vi "PathPlanner_IdealStartingState_Equals.vi"(9 "Other IdealStartingState":T1={"VelocityMPS"=0.0, "Rotation"={"VALUE"=0.0, "COS"=1.0, "SIN"=0.0}, "NotNull"=FALSE} {"Rotation"."SIN" format="%13.4f"; "Rotation"."COS" format="%13.4f"; "Rotation"."VALUE" format="%13.4f"}, 11 "IdealStartingState":T1={"VelocityMPS"=0.0, "Rotation"={"VALUE"=0.0, "COS"=1.0, "SIN"=0.0}, "NotNull"=FALSE} {"Rotation"."SIN" format="%13.4f"; "Rotation"."COS" format="%13.4f"; "Rotation"."VALUE" format="%13.4f"}) -> (3 "Equal":bool)   [LabVIEW 2019, in "PathPlanner24.lvlib"]
doc: "Determines if two Ideal Starting State definitions are equal\n\nInputs:\n -- IdealStartingState - cluster - ideal start state definition\n -- Other IdealStartingState - cluster - ideal start state definition\n\nOutputs:\n -- Equal - boolean - TRUE if both definitions are the same."
uses:
  PathPlanner24.lvlib
  TypeDef/PathPlannerIdealStartingState.ctl
  <vilib>/Rock Robotics/WPI/ThirdParty/JAS_Junk/TrajLib/TypeDef/ROTATION2D.ctl
  <vilib>/Rock Robotics/WPI/ThirdParty/JAS_Junk/TrajLib/Util_CalcDist.vi
  <vilib>/Rock Robotics/WPI/ThirdParty/JAS_Junk/TrajLib/Trajectory_Library.lvlib
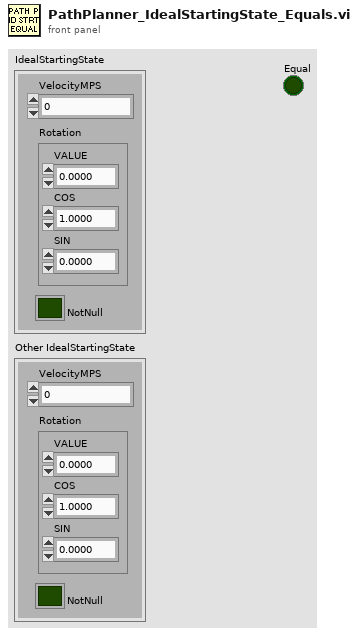
[diagram p1: front panel]
types:
  T1 = typedef "PathPlanner24.lvlib/PathPlannerIdealStartingState.ctl" = cluster{"VelocityMPS":dbl, "Rotation":T2, "NotNull":bool}
  T2 = typedef "Trajectory_Library.lvlib/ROTATION2D.ctl" = cluster{"VALUE":dbl, "COS":dbl, "SIN":dbl}
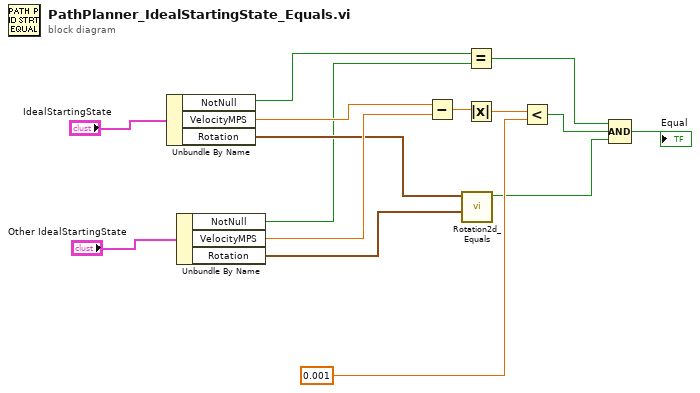
[diagram p0: block diagram]
diagram:
  n1 = Unbundle By Name("IdealStartingState") -> ("NotNull"=w3:bool, "VelocityMPS"=w13:dbl, "Rotation"=w6:T2)
  n2 = Unbundle By Name("Other IdealStartingState") -> ("NotNull"=w2:bool, "VelocityMPS"=w12:dbl, "Rotation"=w5:T2)
  n3 = Subtract(x=w13, y=w12) -> (x-y=w11:dbl)
  n4 = call <vilib>:"Rotation2d_Equals.vi"("other ROTATION"=w5, "in ROTATION"=w6) -> ("Equals"=w4:bool)  [unwired: 9 in]
  n5 = Equal?(x=w3, y=w2) -> (x = y?=w1:bool)
  n6 = Absolute Value(x=w11) -> (abs(x)=w10:dbl)
  n7 = Less?(x=w10, y=0.001) -> (x < y?=w9:bool)
  n8 = Compound Arithmetic op=AND(w1, w9, w4) -> (→"Equal":bool)
